vi "Benchmark Execute.vi"(8 "error in (no error)":errorcluster, 11 "CIFCorePlugin in":refnum<class "CIFCorePlugin.lvclass">) -> (0 "error out":errorcluster, 3 "CIFCorePlugin out":refnum<class "CIFCorePlugin.lvclass">)   [LabVIEW 2021, in "CIFCorePlugin.lvclass"]
doc: "This VI will perform core benchmarks of execute and sleep. These are done together since the standard pattern is sleep, followed by execution. \n\nThis VI should be called at the end of execution (normally the start of housekeeping). This VI will be called automatically at the start of housekeeping unless \"Disable Auto Benchmark\" is configured true for the plugin. \n\nIf \"Skip Sleep\" is configured for the plugn AND multiple sleep/execute operations may occur during the logic step, this can be called manually at the end of each execute operation."
uses:
  CIFCorePlugin.lvclass
  CIFCorePlugin.lvclass/CIFCorePlugin.ctl
  <vilib>/CIF Foundation/CIF Utilities/Statistics/I64/Stats_I64_CIF_U.lvclass/Stats_I64_CIF_U.ctl
  Accessors/Timestamps/Read Execute TS.vi
  Accessors/Timestamps/Read Housekeeping TS.vi
  Accessors/Timestamps/Read Sleep TS.vi
  Accessors/Timestamps/Read Target Wake TS.vi
  <vilib>/CIF Foundation/CIF Utilities/Time/System Time/LabVIEW Time to TAI Time.vi
  <vilib>/CIF Foundation/CIF Utilities/Statistics/I64/X1 minus X0.vi/dfabcf33-0dbc-4041-80a5-3dc0c86d2989.vi
  <vilib>/CIF Foundation/CIF Utilities/Statistics/I64/Cyclic.vi/dfabcf33-0dbc-4041-80a5-3dc0c86d2989.vi
  <vilib>/CIF Foundation/CIF Utilities/Statistics/I64/X1 minus X0.vi/dfabcf33-0dbc-4041-80a5-3dc0c86d2989.vi/9eb60a9a-770f-4d2d-8b3f-8465c267ecc9.vi
  <vilib>/CIF Foundation/CIF Utilities/Statistics/I64/Cyclic.vi/dfabcf33-0dbc-4041-80a5-3dc0c86d2989.vi/9eb60a9a-770f-4d2d-8b3f-8465c267ecc9.vi
  <vilib>/CIF Foundation/CIF Utilities/Time/Time_CIF_U.lvlib
  <vilib>/CIF Foundation/CIF Utilities/Statistics/I64/Stats_I64_CIF_U.lvclass
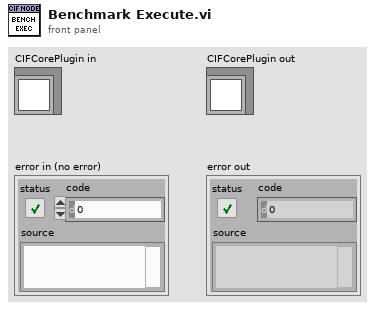
[diagram p1: front panel]
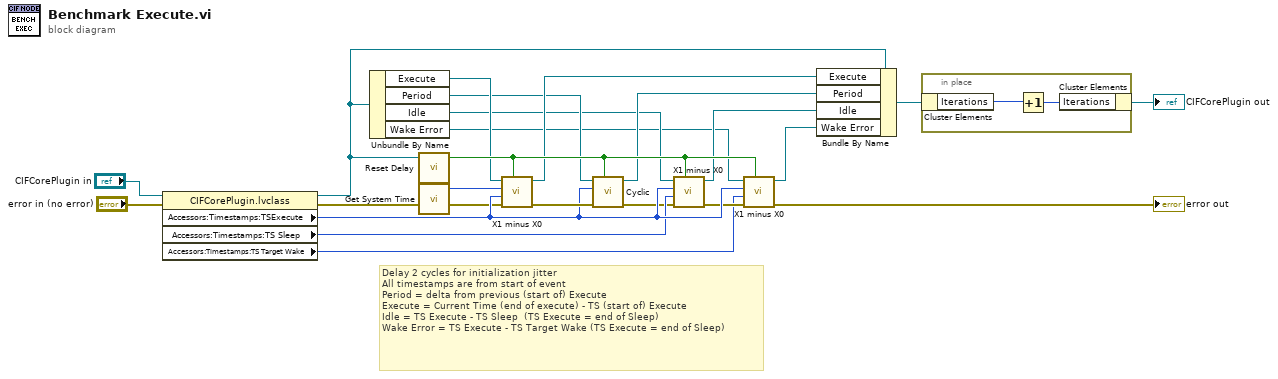
[diagram p0: block diagram]
diagram:
  # "Delay 2 cycles for initialization jitter\nAll timestamps are from start of event\nPeriod = delta from previous (start of) Execute\nExecute = Current Time (end of execute) - TS (start of) Execute\nIdle = TS Execute - TS Sleep  (TS Execute = end of Sleep)\nWake Error = TS Execute - TS Target Wake (TS Execute = end of Sleep)"
  n1 = property class="CIFCorePlugin.lvclass"(reference="CIFCorePlugin in", error in="error in (no error)") -> (reference out=w4:refnum<class "CIFCorePlugin.lvclass">, error out=w5:errorcluster, "Accessors:Timestamps:TSExecute"=w19:i64, "Accessors:Timestamps:TS Sleep"=w9:i64, "Accessors:Timestamps:TS Target Wake"=w10:i64)
  n2 = Unbundle By Name(w4) -> ("Execute"=w20:refnum<class "Stats_I64_CIF_U.lvclass">, "Period"=w18:refnum<class "Stats_I64_CIF_U.lvclass">, "Idle"=w16:refnum<class "Stats_I64_CIF_U.lvclass">, "Wake Error"=w14:refnum<class "Stats_I64_CIF_U.lvclass">)
  n3 = call "Reset Delay.vi"("CIFCorePlugin in"=w4) -> ("Reset"=w23:bool)  [unwired: 3 in]
  n4 = call <vilib>:"Get System Time.vi"() -> ("Time (ns)"=w8:i64)  [unwired: 5 in]
  n5 = call <vilib>:"X1 minus X0.vi"("Reinit"=w23, "error in (no error)"=w5, "X0"=w19, "X1"=w8, "Stats_I64_CIF_U in"=w20) -> ("error out"=w22:errorcluster, "Stats_I64_CIF_U out"=w21:refnum<class "Stats_I64_CIF_U.lvclass">)  [unwired: 5 in]
  n6 = call <vilib>:"Cyclic.vi"("Reinit"=w23, "error in (no error)"=w22, "X"=w19, "Stats_I64_CIF_U in"=w18) -> ("error out"=w3:errorcluster, "Stats_I64_CIF_U out"=w17:refnum<class "Stats_I64_CIF_U.lvclass">)  [unwired: 6 in]
  n7 = call <vilib>:"X1 minus X0.vi"("Reinit"=w23, "error in (no error)"=w3, "X0"=w9, "X1"=w19, "Stats_I64_CIF_U in"=w16) -> ("error out"=w12:errorcluster, "Stats_I64_CIF_U out"=w15:refnum<class "Stats_I64_CIF_U.lvclass">)  [unwired: 5 in]
  n8 = call <vilib>:"X1 minus X0.vi"("Reinit"=w23, "error in (no error)"=w12, "X0"=w10, "X1"=w19, "Stats_I64_CIF_U in"=w14) -> ("error out"=→"error out":errorcluster, "Stats_I64_CIF_U out"=w13:refnum<class "Stats_I64_CIF_U.lvclass">)  [unwired: 5 in]
  n9 = Bundle By Name(cluster=w4, "Execute"=w21, "Period"=w17, "Idle"=w15, "Wake Error"=w13) -> (w2:refnum<class "CIFCorePlugin.lvclass">)
  n10 = in-place {
    n11 = in-place-cluster #1(w2) -> ("Iterations"=w24:i64)
    n12 = Increment(x=w24) -> (x+1=w25:i64)
    n13 = in-place-cluster #1("Iterations"=w25) -> (→"CIFCorePlugin out":refnum<class "CIFCorePlugin.lvclass">)
  }
